vi "PH_PSDBWriter.Wrap PSDB Dataset.vi"(0 "Version":i32, 1 "2D data Input":T1[](array[typedef]), 2 "Boolean Input":T3[](array[typedef]), 3 "Image Input":T4[](array[typedef]), 4 "Numeric Input":T6[](array[typedef]), 5 "String Input":T8[](array[typedef])) -> (16 "PSDB Dataset":T7)   [LabVIEW 2014, in "PH_PSDBWriter.lvlib"]
doc: "This VI wraps all data for a PSDB Dataset."
uses:
  PH_PSDBWriter.lvlib
  PH_PSDBWriter.PSDB Dataset.ctl
  PH_PSDBWriter.2D dataset.ctl
  User/Eisenbarth/psdb_lv/PSDB_AxisDescription.ctl
  PH_PSDBWriter.Boolean dataset.ctl
  PH_PSDBWriter.Image dataset.ctl
  <vilib>/vision/Image Controls.llb/IMAQ Image.ctl
  PH_PSDBWriter.Numeric dataset.ctl
  PH_PSDBWriter.String dataset.ctl
  User/Eisenbarth/psdb_lv/PSDB.lvlib
panel:
  in  "PSDB Dataset in":T7
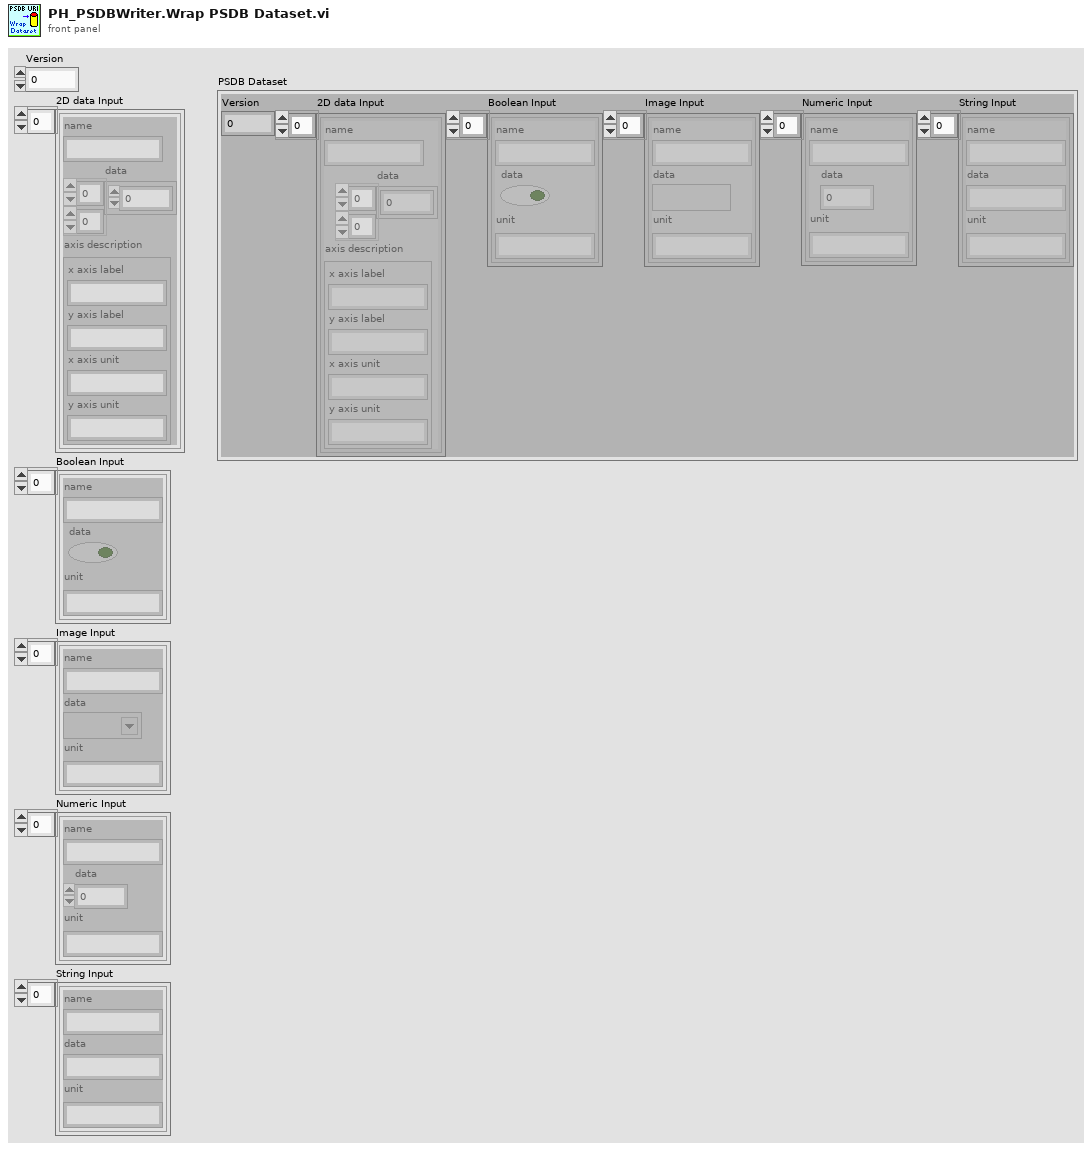
[diagram p1: front panel]
types:
  T1 = typedef "PH_PSDBWriter.lvlib/PH_PSDBWriter.2D dataset.ctl" = cluster{"name":string, "data":dbl[][], "axis description":T2}
  T2 = typedef "PSDB.lvlib/PSDB_AxisDescription.ctl" = cluster{"x axis label":string, "y axis label":string, "x axis unit":string, "y axis unit":string}
  T3 = typedef "PH_PSDBWriter.lvlib/PH_PSDBWriter.Boolean dataset.ctl" = cluster{"name":string, "data":bool, "unit":string}
  T4 = typedef "PH_PSDBWriter.lvlib/PH_PSDBWriter.Image dataset.ctl" = cluster{"name":string, "data":T5, "unit":string}
  T5 = typedef "IMAQ Image.ctl" = refnum<image>
  T6 = typedef "PH_PSDBWriter.lvlib/PH_PSDBWriter.Numeric dataset.ctl" = cluster{"name":string, "data":dbl, "unit":string}
  T7 = typedef "PH_PSDBWriter.lvlib/PH_PSDBWriter.PSDB Dataset.ctl" = cluster{"Version":i32, "2D data Input":T1[], "Boolean Input":T3[], "Image Input":T4[], "Numeric Input":T6[], "String Input":T8[]}
  T8 = typedef "PH_PSDBWriter.lvlib/PH_PSDBWriter.String dataset.ctl" = cluster{"name":string, "data":string, "unit":string}
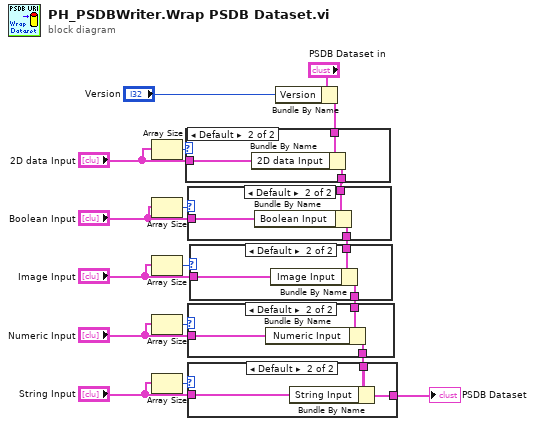
[diagram p0: block diagram]
diagram:
  n1 = Array Size(array="2D data Input") -> (size(s)=w15:i32)
  n2 = Array Size(array="Boolean Input") -> (size(s)=w9:i32)
  n3 = Array Size(array="Image Input") -> (size(s)=w7:i32)
  n4 = Array Size(array="Numeric Input") -> (size(s)=w6:i32)
  n5 = Array Size(array="String Input") -> (size(s)=w5:i32)
  n6 = Bundle By Name(cluster="PSDB Dataset in", "Version"="Version") -> (w16:T7)
  n7 = case shown="Default" w15 {
    tunnel: [w19 w22] -> w13
    tunnel: w16 -> [w19 w21]
    tunnel: "2D data Input" -> [_ w20]
    frame 0 {
    }
    frame Default {
      n8 = Bundle By Name(cluster=w21, "2D data Input"=w20) -> (w22:T7)
    }
  }
  n9 = case shown="Default" w9 {
    tunnel: [w23 w26] -> w12
    tunnel: w13 -> [w23 w25]
    tunnel: "Boolean Input" -> [_ w24]
    frame 0 {
    }
    frame Default {
      n10 = Bundle By Name(cluster=w25, "Boolean Input"=w24) -> (w26:T7)
    }
  }
  n11 = case shown="Default" w7 {
    tunnel: [w27 w30] -> w11
    tunnel: w12 -> [w27 w29]
    tunnel: "Image Input" -> [_ w28]
    frame 0 {
    }
    frame Default {
      n12 = Bundle By Name(cluster=w29, "Image Input"=w28) -> (w30:T7)
    }
  }
  n13 = case shown="Default" w6 {
    tunnel: [w31 w34] -> w10
    tunnel: w11 -> [w31 w33]
    tunnel: "Numeric Input" -> [_ w32]
    frame 0 {
    }
    frame Default {
      n14 = Bundle By Name(cluster=w33, "Numeric Input"=w32) -> (w34:T7)
    }
  }
  n15 = case shown="Default" w5 {
    tunnel: [w35 w38] -> w1
    tunnel: w10 -> [w35 w37]
    tunnel: "String Input" -> [_ w36]
    frame 0 {
    }
    frame Default {
      n16 = Bundle By Name(cluster=w37, "String Input"=w36) -> (w38:T7)
    }
  }
  "PSDB Dataset" <- w1
